vi "WacomConfig.vi"(2 "Mode":enum16{"Load", "Create"}(ring)=enum."Create") -> ()   [LabVIEW 2011]
panel:
  in  "ConfigFile":path
  out "StandardOutput":string
  out "StandardError":string
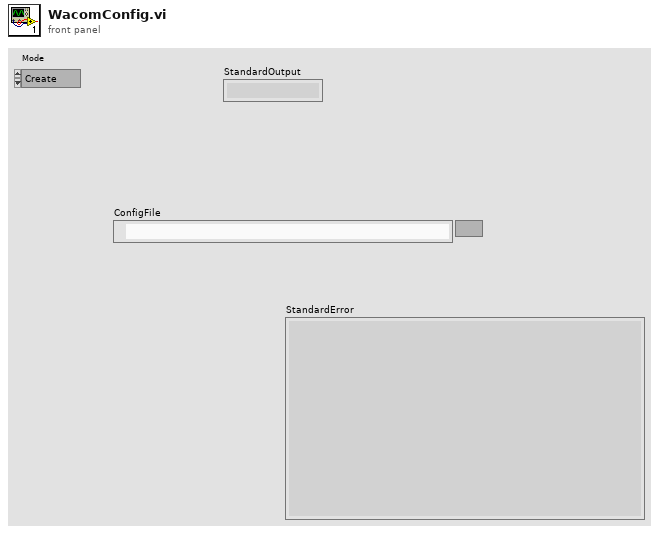
[diagram p1: front panel]
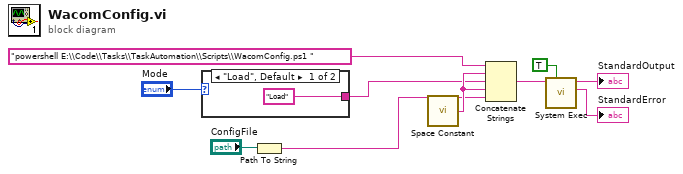
[diagram p0: block diagram]
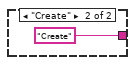
[diagram p2: hidden frame]
diagram:
  n1 = case shown="\"Load\", Default" "Mode" {
    tunnel: ["Load" "Create"] -> w4
    frame "Load", Default {
    }
    frame "Create" {
    }
  }
  n2 = Path To String(path="ConfigFile") -> (string=w1:string)
  n3 = call <vilib>:"Space Constant.vi"() -> ("String"=w9:string)
  n4 = Concatenate Strings("powershell E:\\Code\\Tasks\\TaskAutomation\\Scripts\\WacomConfig.ps1 ", w9, w4, w9, w1) -> (w6:string)
  n5 = call <vilib>:"System Exec.vi"("wait until completion? (T)"=TRUE, "command line"=w6) -> ("standard error"=→"StandardError":string, "standard output"=→"StandardOutput":string)  [unwired: 6 in, 2 out]
